vi "等分取数据.vi"(0 "Max":dbl, 1 "MIN":dbl, 3 "num":i32) -> (7 "数据点":dbl[](array[numeric]))   [LabVIEW 2010]
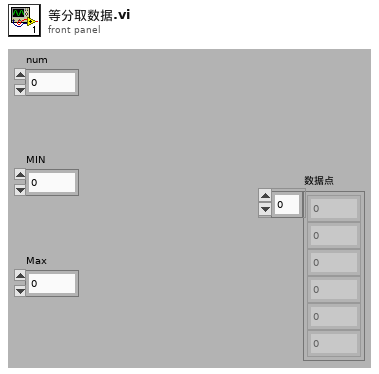
[diagram p1: front panel]
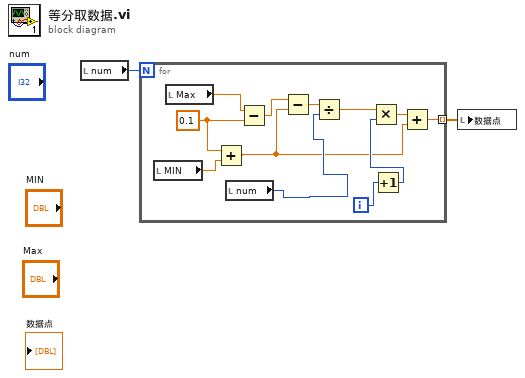
[diagram p0: block diagram]
diagram:
  n1 = local read "num"() -> (w1:i32)
  n2 = for {
    N: w1 -> [_]
    tunnel: [w11] -> w2 mode=indexing
    i -> [w10]
    w5 = 0.1
    n3 = local read "MIN"() -> (w4:dbl)
    n4 = local read "Max"() -> (w7:dbl)
    n5 = Add(x=w5, y=w4) -> (x+y=w3:dbl)
    n6 = local read "num"() -> (w8:i32)
    n7 = Subtract(x=w7, y=w5) -> (x-y=w6:dbl)
    n8 = Subtract(x=w6, y=w3) -> (x-y=w14:dbl)
    n9 = Divide(x=w14, y=w8) -> (x/y=w13:dbl)
    n10 = Increment(x=w10) -> (x+1=w9:i32)
    n11 = Multiply(x=w13, y=w9) -> (x*y=w12:dbl)
    n12 = Add(x=w12, y=w3) -> (x+y=w11:dbl)
  }
  n13 = local write "数据点"(w2) -> ()
